vi "FTW-STR-UTF16.vi"(0 "Input":string, 1 "Direction":T1) -> (2 "Output":string)   [LabVIEW 2013]
uses:
  Core/src/String/FTW-STR-EncodingDirection.ctl
panel:
  # "Inputs"
  # "Outputs"
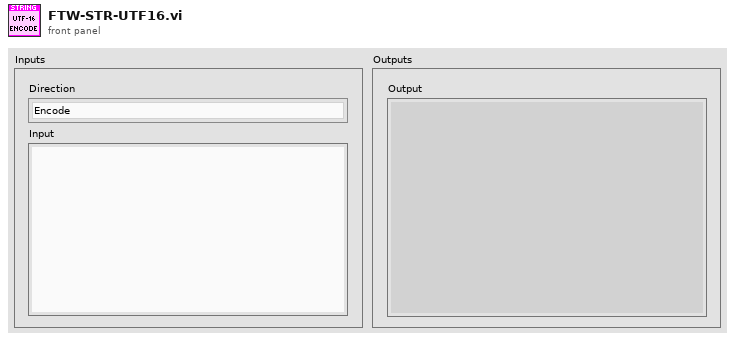
[diagram p1: front panel]
types:
  T1 = typedef "FTW-STR-EncodingDirection.ctl" = enum16{"Encode", "Decode"}
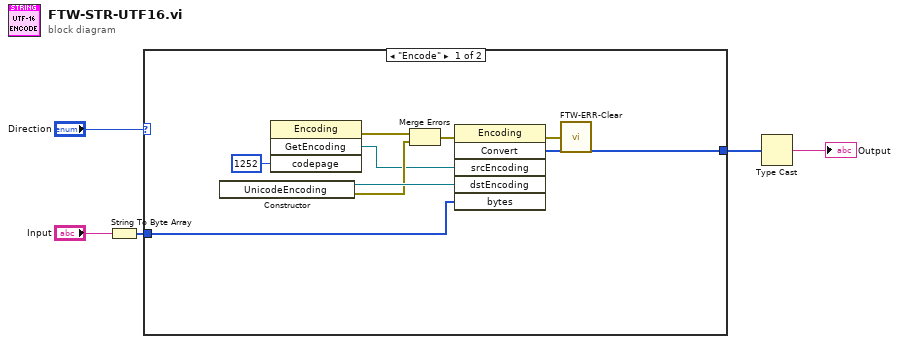
[diagram p0: block diagram]
diagram:
  n1 = String To Byte Array(string="Input") -> (unsigned byte array=w3:u8[])
  n2 = case shown="\"Encode\"" "Direction" {
    tunnel: [w13 w15] -> w4
    tunnel: w3 -> [w12 w15]
    frame "Encode" {
      n3 = constructor class="UnicodeEncoding"() -> (reference out=w14:refnum<k24>, error out=w9:errorcluster)  [unwired: 3 in, 1 out]
      n4 = invoke class="Encoding" method="GetEncoding"("codepage"=1252) -> (error out=w6:errorcluster, "GetEncoding"=w7:refnum<k24>)  [unwired: 3 in, 2 out]
      n5 = Merge Errors(w6, w9) -> (w11:errorcluster)
      n6 = invoke class="Encoding" method="Convert"(error in=w11, "srcEncoding"=w7, "dstEncoding"=w14, "bytes"=w12) -> (error out=w10:errorcluster, "Convert"=w13:u8[])  [unwired: 2 in, 4 out]
      n7 = call "FTW-ERR-Clear.vi"("error to snuff"=w10) -> ()  [unwired: 1 out]
    }
    frame "Decode" {
      # "Not yet implemented."
    }
  }
  n8 = Type Cast(x=w4) -> (*(type *) &x=→"Output":string)  [unwired: 1 in]
